vi "Find Rotation Center.vi"() -> ()   [LabVIEW 2021, in "Test VIs.lvclass"]
uses:
  Test VIs/Test VIs.lvclass
  Classes/Routine/Routine Enum.ctl
  Classes/Workspace/Workspace.ctl
  Classes/Routine/Routine.lvclass
  Classes/Controller/Controller.lvclass
  Classes/Workspace/Fixture.lvclass
panel:
  out "Offset":dbl[](array[numeric])
  in  "Direction":enum16{"Clockwise", "Counter Clockwise"}(ring)
  in  "New Fiducial":dbl[](array[numeric])
  in  "Submit":bool
  in  "Go":bool
  in  "Original Fiducial":dbl[](array[numeric])
  in  "Input Rotation Center":dbl[](array[numeric])
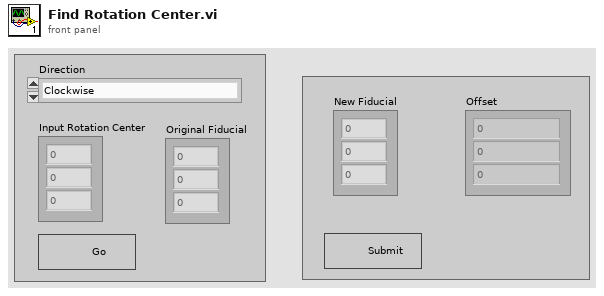
[diagram p1: front panel]
types:
  T1 = typedef "Controller.lvclass/Controllers.ctl" = cluster{"I-O.lvclass":refnum<class "I-O.lvclass">, "Gantry":refnum<k24>, "Dispenser":refnum<visa-resource-name>}
  T2 = typedef "Fixture.lvclass/Workspace.ctl" = cluster{"XYZTheta":dbl[], "Workspace Valve":i32, "Workspace Sensor":i32, "Tray Number":i32, "Position":i32, "Assembly Type":string, "Numeric":dbl, "First Pos":i32}
  T3 = typedef "Routine.lvclass/Routine Enum.ctl" = enum16{"Primary Pick Up", "Secondary Pick Up", "Put Down All", "Secure Syringe", "Release Syringe", "Dispense Epoxy", "Pick Up All", "Put Down Secondary", "Full Assembly"}
  T4 = typedef "File Paths.ctl" = cluster{"Glue Pattern Folder":path, "Carrier Tray Folder":path, "Pick Up Tool Fixture Folder":path, "Components Folder":path, "Bellows Tool Offset.txt":path, "Pick Up Tool Offset.txt":path, "Dispense Tip Offset.txt":path, "Log Files":path, "Gantry Assembly Map.txt":path, "Syringe and offset map.txt":path, "Controllers Folder":path, "Local dbase config":path}
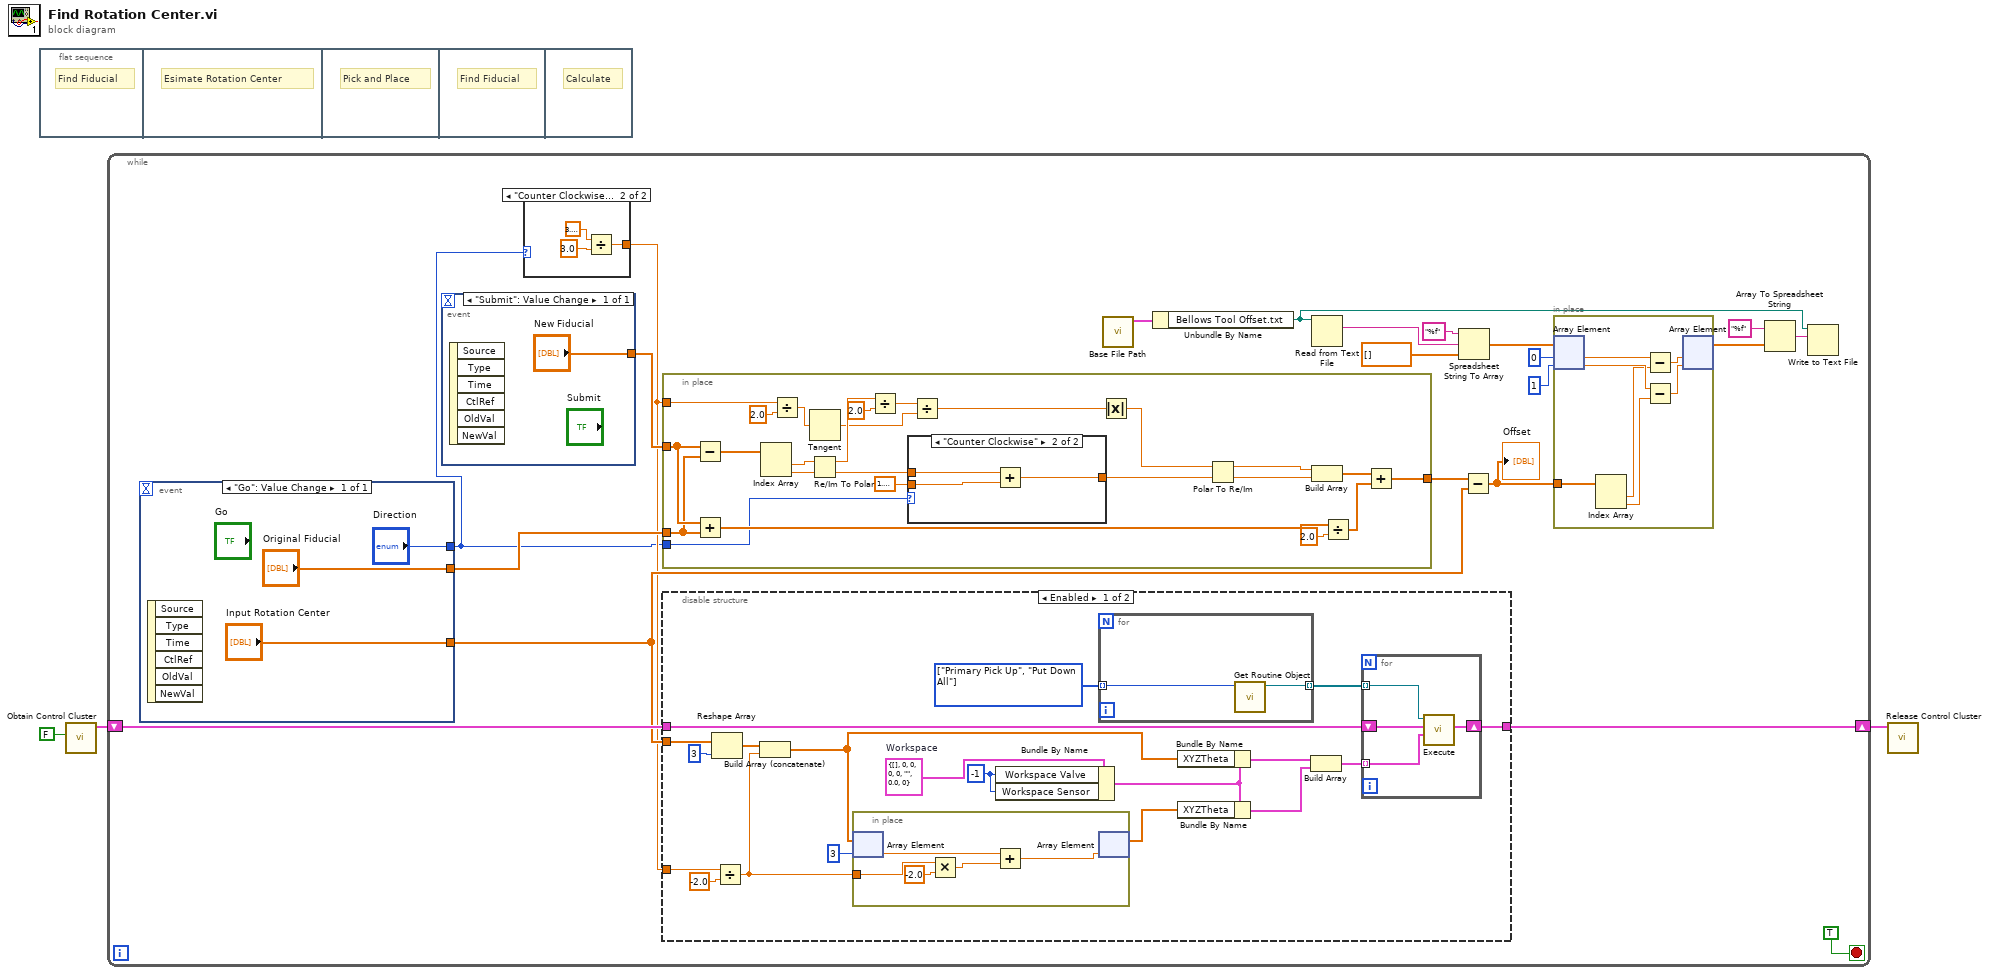
[diagram p0: block diagram]
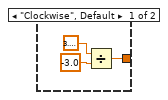
[diagram p3: hidden frame]
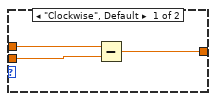
[diagram p4: hidden frame]
diagram:
  n1 = flat-sequence {
    frame #0 {
      # "Find Fiducial"
    }
    frame #1 {
      # "Esimate Rotation Center"
    }
    frame #2 {
      # "Pick and Place"
    }
    frame #3 {
      # "Find Fiducial"
    }
    frame #4 {
      # "Calculate"
    }
  }
  n2 = call "Obtain Control Cluster.vi"("Dispense"=FALSE) -> ("Control Out"=w2:T1)  [unwired: 9 in, 1 out]
  n3 = while {
    shift-right: [w23] -> w1
    shift-left: w2 -> [w24]
    stop <- TRUE stop-if-true
    n4 = event shown="[0] \"Go\": Value Change" {
      selector: _ -> [_]
      dyn-events: _ -> [_]
      timeout: _ -> [_]
      tunnel: ["Input Rotation Center"] -> w11
      tunnel: ["Original Fiducial"] -> w10
      tunnel: ["Direction"] -> w6
      event "Go": Value Change {
        n5 = event-data() -> ()  [unwired: 1 in, 6 out]
      }
    }
    n6 = event shown="[0] \"Submit\": Value Change" {
      selector: _ -> [_]
      dyn-events: _ -> [_]
      timeout: _ -> [_]
      tunnel: ["New Fiducial"] -> w9
      event "Submit": Value Change {
        n7 = event-data() -> ()  [unwired: 1 in, 6 out]
      }
    }
    n8 = case shown="\"Counter Clockwise\"" w6 {
      tunnel: [w56 w59] -> w7
      frame "Clockwise", Default {
        n9 = Divide(x=3.141592653589793, y=-3.0) -> (x/y=w56:dbl)
      }
      frame "Counter Clockwise" {
        n10 = Divide(x=3.141592653589793, y=3.0) -> (x/y=w59:dbl)
      }
    }
    n11 = in-place {
      in-place-border: w10 -> [w87]
      in-place-border: w9 -> [w88]
      in-place-border: [w80] -> w22
      in-place-border: w7 -> [w77]
      in-place-border: w6 -> [w78]
      n12 = Subtract(x=w88, y=w87) -> (x-y=w97:dbl[])
      n13 = Add(x=w88, y=w87) -> (x+y=w86:dbl[])
      n14 = Index Array(array=w97) -> (element #1=w96:dbl, element #2=w95:dbl)  [unwired: 2 in]
      n15 = Divide(x=w77, y=2.0) -> (x/y=w75:dbl)
      n16 = Tangent(1:w75) -> (0:w91:dbl)
      n17 = Re/Im To Polar(2:w95, 3:w96) -> (0:w79:dbl, 1:w93:dbl)
      n18 = Divide(x=w93, y=2.0) -> (x/y=w92:dbl)
      n19 = case shown="\"Counter Clockwise\"" w78 {
        tunnel: w79 -> [w100 w103]
        tunnel: 1.5707963267948966 -> [w99 w102]
        tunnel: [w98 w101] -> w89
        frame "Clockwise", Default {
          n20 = Subtract(x=w100, y=w99) -> (x-y=w98:dbl)
        }
        frame "Counter Clockwise" {
          n21 = Add(x=w103, y=w102) -> (x+y=w101:dbl)
        }
      }
      n22 = Divide(x=w92, y=w91) -> (x/y=w74:dbl)
      n23 = Absolute Value(x=w74) -> (abs(x)=w73:dbl)
      n24 = Polar To Re/Im(2:w89, 3:w73) -> (0:w84:dbl, 1:w85:dbl)
      n25 = Build Array(w85, w84) -> (w83:dbl[])
      n26 = Divide(x=w86, y=2.0) -> (x/y=w81:dbl[])
      n27 = Add(x=w83, y=w81) -> (x+y=w80:dbl[])
    }
    n28 = disable-structure shown="Enabled" {
      disable-tunnel: w24 -> [w43 w55]
      disable-tunnel: [w42 w55] -> w23
      disable-tunnel: w11 -> [w30 _]
      disable-tunnel: w7 -> [w33 _]
      frame Enabled {
        w27 = -1 ("Workspace Valve")
        w26 = T2 {"XYZTheta"=[], "Workspace Valve"=0, "Workspace Sensor"=0, "Tray Number"=0, "Position"=0, "Assembly Type"="", "Numeric"=0.0, "First Pos"=0}  # Workspace
        w40 = T3[] [enum."Primary Pick Up", enum."Put Down All"] items=["Primary Pick Up", "Secondary Pick Up", "Put Down All", "Secure Syringe", "Release Syringe", "Dispense Epoxy", "Pick Up All", "Put Down Secondary", "Full Assembly"]
        n29 = Reshape Array(w30, 3 ("dimension size")) -> (w28:dbl[])
        n30 = Divide(x=w33, y=-2.0) -> (x/y=w31:dbl)
        n31 = Build Array (concatenate)(w28, w31) -> (w39:dbl[])
        n32 = in-place {
          in-place-border: w31 -> [w47]
          n33 = in-place-array #1(w39, 3) -> (w48:dbl)
          n34 = Multiply(x=w47, y=-2.0) -> (x*y=w45:dbl)
          n35 = Add(x=w48, y=w45) -> (x+y=w44:dbl)
          n36 = in-place-array #1(w44) -> (w37:dbl[])  [unwired: 1 out]
        }
        n37 = Bundle By Name(cluster=w26, "Workspace Valve"=w27, "Workspace Sensor"=w27) -> (w25:T2)
        n38 = for {
          tunnel: [w50] -> w41 mode=indexing
          tunnel: w40 -> [w49] mode=indexing
          n39 = call "Get Routine Object.vi"("Routine"=w49) -> ("Routine out"=w50:refnum<class "Routine.lvclass">)  [unwired: 9 in, 1 out]
        }
        n40 = Bundle By Name(cluster=w25, "XYZTheta"=w39) -> (w36:T2)
        n41 = Bundle By Name(cluster=w25, "XYZTheta"=w37) -> (w34:T2)
        n42 = Build Array(w36, w34) -> (w35:T2[])
        n43 = for {
          shift-right: [w53] -> w42
          shift-left: w43 -> [w54]
          tunnel: w41 -> [w52] mode=indexing
          tunnel: w35 -> [w51] mode=indexing
          n44 = call-dynamic "Execute.vi"("Workspace"=w51, "Control In"=w54, "Routine in"=w52) -> ("Control Out"=w53:T1)  [unwired: 6 in, 2 out]
        }
      }
      frame Disabled {
      }
    }
    n45 = call "Base File Path.vi"() -> ("Paths Out"=w21:T4)  [unwired: 11 in]
    n46 = Unbundle By Name(w21) -> ("Bellows Tool Offset.txt"=w8:path)
    n47 = Read from Text File(file (use dialog)=w8) -> (text=w20:string)  [unwired: 3 in, 3 out]
    n48 = Spreadsheet String To Array(format string="%f", spreadsheet string=w20, array type (2D Dbl)=dbl[] []) -> (array=w18:dbl[])  [unwired: 1 in]
    n49 = Subtract(x=w22, y=w11) -> (x-y=w5:dbl[])
    "Offset" <- w5
    n50 = in-place {
      in-place-border: w5 -> [w72]
      n51 = in-place-array #2(w18, 0, 1) -> (w71:dbl, w70:dbl)
      n52 = Index Array(array=w72) -> (element #1=w69:dbl, element #2=w68:dbl)  [unwired: 2 in]
      n53 = Subtract(x=w71, y=w69) -> (x-y=w66:dbl)
      n54 = Subtract(x=w70, y=w68) -> (x-y=w67:dbl)
      n55 = in-place-array #2(w66, w67) -> (w17:dbl[])  [unwired: 2 out]
    }
    n56 = Array To Spreadsheet String(array=w17, 3:"%f" ("format string")) -> (spreadsheet string=w15:string)  [unwired: 1 in]
    n57 = Write to Text File(file (use dialog)=w8, text=w15) -> ()  [unwired: 2 in, 3 out]
  }
  n58 = call "Release Control Cluster.vi"("output cluster"=w1) -> ()  [unwired: 11 in]
